vi "RenameFrame__slk_mt.vi"(8 "error in (no error)":errorcluster, 9 "old frame name":string, 10 "new frame name":string, 11 "case model in":refnum<class "CaseModel__slk_mt.lvclass">) -> (0 "error out":errorcluster, 3 "case model out":refnum<class "CaseModel__slk_mt.lvclass">)   [LabVIEW 2015, in "CaseModel__slk_mt.lvclass"]
doc: "Renames frame name."
uses:
  CaseModel__slk_mt.lvclass
panel:
  # "RenameFrame__slk_mt.vi\nRenames frame name.\n\nNOTICE -- YOU MUST LEAVE THIS NOTICE IN PLACE.\n\nCopyright (c) 2011, LIANG LIU Shawn.Liu.cn@gmail.com\nAll rights reserved.\n\nRedistribution and use in source and binary forms, with or without modification, are permitted provided that the following conditions are met:\n-Redistributions of source code must retain the above copyright notice, this list of conditions and the following disclaimer.\n-Redistributions in binary form must reproduce the above copyright notice, this list of conditions and the following disclaimer in the documentation and/or other materials provided with the distribution.\n-Neither the name of the eLp nor the names of its contributors may be used to endorse or promote products derived from this software without specific prior written permission.\n\nTHIS SOFTWARE IS PROVIDED BY THE COPYRIGHT HOLDERS AND CONTRIBUTORS \"AS IS\" AND ANY EXPRESS OR IMPLIED WARRANTIES, INCLUDING, BUT NOT LIMITED TO, THE IMPLIED WARRANTIES OF MERCHANTABILITY AND FITNESS FOR A PARTICULAR PURPOSE ARE DISCLAIMED. IN NO EVENT SHALL THE COPYRIGHT HOLDER OR CONTRIBUTORS BE LIABLE FOR ANY DIRECT, INDIRECT, INCIDENTAL, SPECIAL, EXEMPLARY, OR CONSEQUENTIAL DAMAGES (INCLUDING, BUT NOT LIMITED TO, PROCUREMENT OF SUBSTITUTE GOODS OR SERVICES; LOSS OF USE, DATA, OR PROFITS; OR BUSINESS INTERRUPTION) HOWEVER CAUSED AND ON ANY THEORY OF LIABILITY, WHETHER IN CONTRACT, STRICT LIABILITY, OR TORT (INCLUDING NEGLIGENCE OR OTHERWISE) ARISING IN ANY WAY OUT OF THE USE OF THIS SOFTWARE, EVEN IF ADVISED OF THE POSSIBILITY OF SUCH DAMAGE."
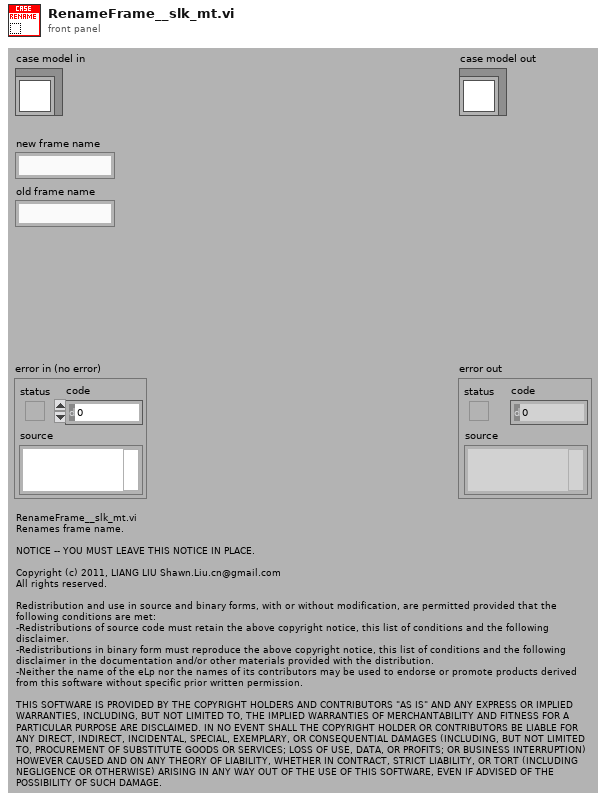
[diagram p1: front panel]
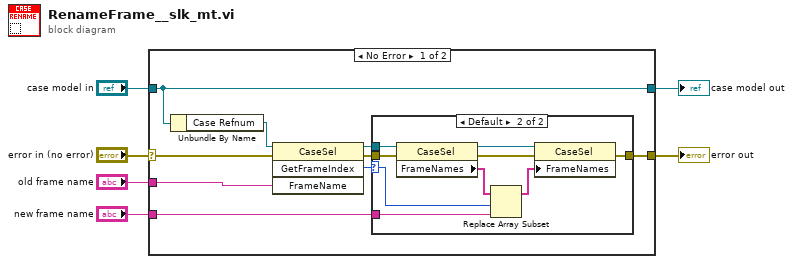
[diagram p0: block diagram]
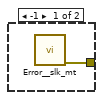
[diagram p2: hidden frame]
diagram:
  n1 = case shown="No Error" "error in (no error)" {
    selector: "error in (no error)" -> [w7 w27]
    tunnel: [w12 w27] -> w5
    tunnel: [w10 w26] -> w3
    tunnel: "case model in" -> [w10 w26]
    tunnel: "old frame name" -> [w9 _]
    tunnel: "new frame name" -> [w8 _]
    frame No Error {
      n2 = Unbundle By Name(w10) -> ("Case Refnum"=w15:refnum<vi>)
      n3 = invoke class="CaseSel" method="GetFrameIndex"(reference=w15, error in=w7, "FrameName"=w9) -> (reference out=w14:refnum<vi>, error out=w13:errorcluster, "GetFrameIndex"=w11:i32)  [unwired: 1 in, 1 out]
      n4 = case shown="Default" w11 {
        selector: w11 -> [_ w19]
        tunnel: w14 -> [_ w20]
        tunnel: w13 -> [_ w17]
        tunnel: w8 -> [_ w18]
        tunnel: [w16 w21] -> w12
        frame -1 {
          n5 = call "Error__slk_mt.vi"() -> ("error out"=w16:errorcluster)  [unwired: 11 in]
        }
        frame Default {
          n6 = property class="CaseSel"(reference=w20, error in=w17) -> (reference out=w24:refnum<vi>, error out=w23:errorcluster, "FrameNames"=w25:string[])
          n7 = Replace Array Subset(array=w25, new element=w18, index=w19) -> (w22:string[])
          n8 = property class="CaseSel"(reference=w24, error in=w23, "FrameNames"=w22) -> (error out=w21:errorcluster)  [unwired: 1 out]
        }
      }
    }
    frame Error {
    }
  }
  "error out" <- w5
  "case model out" <- w3
